vi "Configure.vi"(6 "GridSize":u32, 7 "Mode":u32, 8 "error in (no error)":errorcluster, 9 "Recording Settings":T1, 11 "AODAcq in":refnum<class "AODAcq.lvclass">) -> (0 "error out":errorcluster, 3 "AODAcq out":refnum<class "AODAcq.lvclass">)   [LabVIEW 2011, in "AODAcq.lvclass"]
uses:
  AODAcq.lvclass
  AODAcq.lvclass/AODAcq.ctl
  <instrlib>/niHWS/nihws.llb/niHWS Group String Attribute ID.ctl
  <instrlib>/niHWS/nihws.llb/niHWS Open File Permissions ID.ctl
  <vilib>/Utility/error.llb/Error Cluster From Error Code.vi
  Program Files/National Instruments/LabVIEW 2011/Targets/NI/FPGA/StockFPGA_IntfPrivate/ScriptTemplates/StockFPGA_PlugInRead32.vi
  <vilib>/rvi/errors/niLvFpgaAdjustHostInterfaceError.vi
  <instrlib>/niHWS/nihws.llb/niHWS Write Analog I16.vi
  <vilib>/rvi/interface/nirviReadWriteControl/nirviReadWriteControl.xnode
  FPGA_Control/AODRef.ctl
  FPGA_Control/FPGA Bitfiles/AODControl_FPGATarget_5751Acquire_F1CF9257.lvbitx
  FPGA_Control/AOD Control (FPGA).vi
  NiFpgaLv.dll
  <vilib>/FPGAPlugInAG/PXIe-7965R/niLvFpga_Read32_PXIe-7965R.vi
  <vilib>/rvi/interface/nirviReadWriteControl/niFpgaRWControlAccessTimeoutTemplate.vi
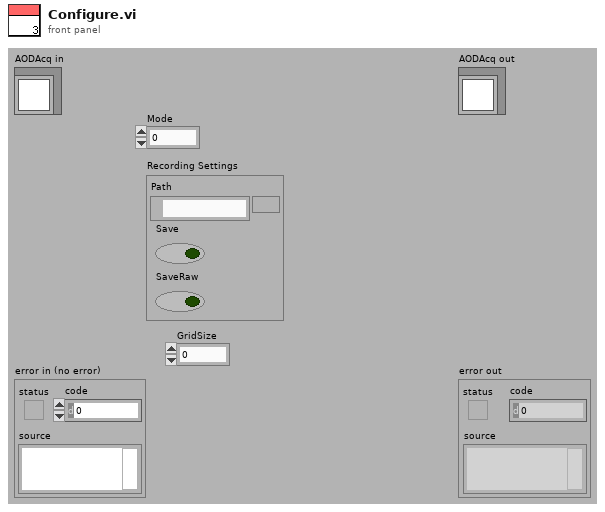
[diagram p1: front panel]
types:
  T1 = cluster{"Path":path, "Save":bool, "SaveRaw":bool}
  T2 = typedef "niHWS Open File Permissions ID.ctl" = enum32{"Read Only", "Read/Write Existing", "Read/Write/Create New", "Read/Write/Create New Always"}
  T3 = typedef "AODRef.ctl" = refnum<k20>
  T4 = typedef "niHWS Group String Attribute ID.ctl" = enum32{"Note", "Technician", "Project", "Timestamp"}
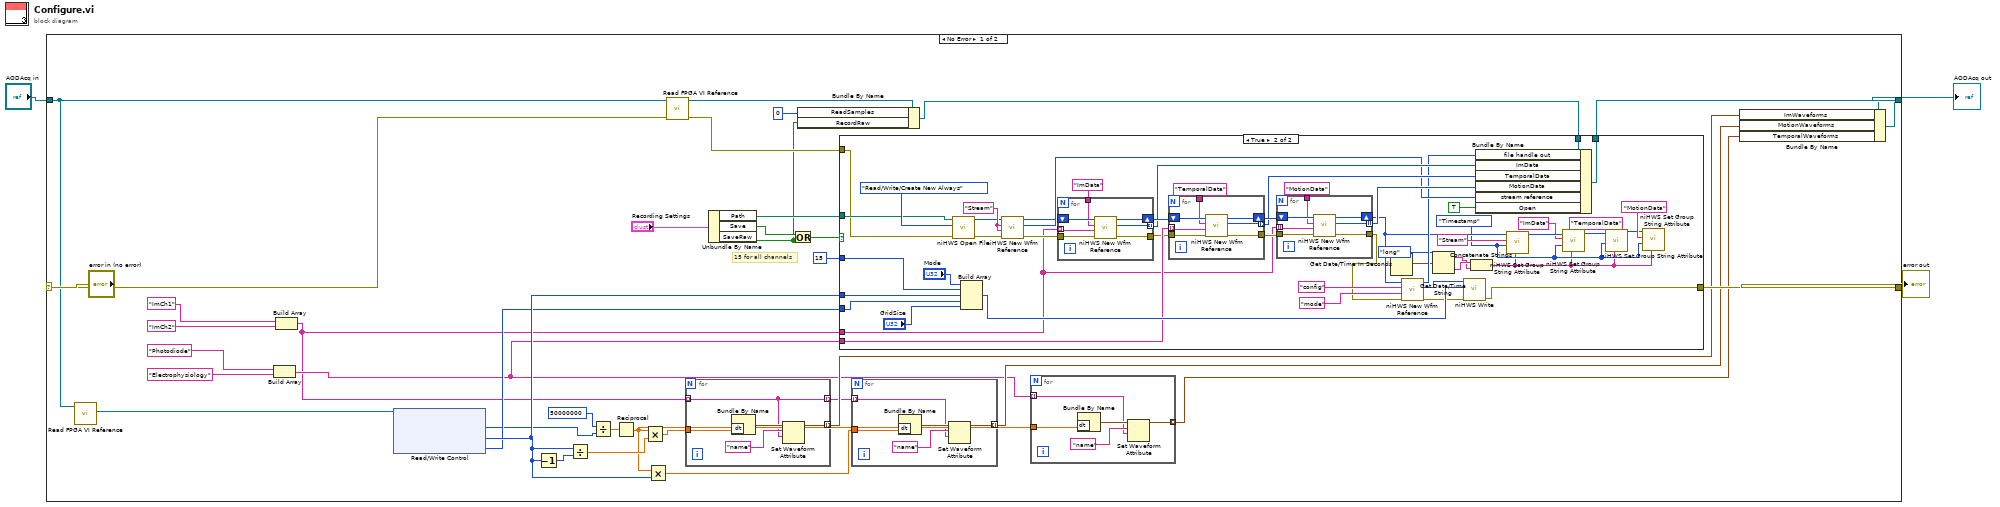
[diagram p0: block diagram]
diagram:
  n1 = case shown="No Error" "error in (no error)" {
    selector: "error in (no error)" -> [w11 w131]
    tunnel: [w36 w131] -> w3
    tunnel: [w26 w130] -> w1
    tunnel: "AODAcq in" -> [w12 w130]
    frame No Error {
      # "15 for all channels"
      n2 = call-dynamic "Read FPGA VI Reference.vi"("AODAcq in"=w12) -> ("FPGA VI Reference"=w29:T3)  [unwired: 8 in, 2 out]
      n3 = Build Array("Photodiode", "Electrophysiology") -> (w10:string[])
      n4 = Build Array("ImCh1", "ImCh2") -> (w9:string[])
      n5 = xnode "Read/Write Control"("FPGA VI Reference In"=w29) -> ("Setup.Downsample"=w5:u32, "Scan.Motion Increment"=w14:u32, "Scan.NumMotionPoints"=w13:u32)  [unwired: 1 in, 2 out]
      n6 = Decrement(x=w14) -> (x-1=w21:u32)
      n7 = Divide(x=w14, y=w21) -> (x/y=w20:dbl)
      n8 = Divide(x=50000000, y=w5) -> (x/y=w31:dbl)
      n9 = Reciprocal(x=w31) -> (1/x=w19:dbl)
      n10 = Multiply(x=w19, y=w20) -> (x*y=w22:dbl)
      n11 = Multiply(x=w19, y=w14) -> (x*y=w18:dbl)
      n12 = call-dynamic "Read FPGA VI Reference.vi"("error in (no error)"=w11, "AODAcq in"=w12) -> ("error out"=w24:errorcluster, "AODAcq out"=w25:refnum<class "AODAcq.lvclass">)  [unwired: 7 in, 1 out]
      n13 = for {
        tunnel: w9 -> [w51] mode=indexing
        tunnel: w22 -> [w55]
        tunnel: [w52] -> w28 mode=indexing
        tunnel: [w51] -> w17 mode=indexing
        n14 = Bundle By Name("dt"=w55) -> (w54:waveform(dbl))  [unwired: 1 in]
        n15 = Set Waveform Attribute(5:w51, 6:"name" ("name"), 7:w54) -> (3:w52:waveform(dbl))  [unwired: 1 in, 2 out]
      }
      n16 = Unbundle By Name("Recording Settings") -> ("Path"=w39:path, "Save"=w40:bool, "SaveRaw"=w23:bool)
      n17 = Or(x=w40, y=w23) -> (x .or. y?=w37:bool)
      n18 = Bundle By Name(cluster=w25, "ReadSamples"=u64 0, "RecordRaw"=w23) -> (w34:refnum<class "AODAcq.lvclass">)
      n19 = case shown="True" w37 {
        tunnel: w39 -> [_ w99]
        tunnel: w34 -> [w57 w95]
        tunnel: [w57 w94] -> w27
        tunnel: w24 -> [w56 w98]
        tunnel: [w56 w78] -> w36
        tunnel: w9 -> [_ w85]
        tunnel: w10 -> [_ w90]
        tunnel: w14 -> [_ w75]
        tunnel: w13 -> [_ w76]
        tunnel: u32 15 -> [_ w74]
        frame False {
        }
        frame True {
          w60 = niHWS_Group_String_Attribute_ID."Timestamp" ("attribute ID")
          w105 = "Stream" ("group name (empty)")
          n20 = call <instrlib>:"niHWS Open File.vi"("error in (no error)"=w98, "permissions (0:read only)"=niHWS_Open_File_Permissions_ID."Read/Write/Create New Always", "file path"=w99) -> ("error out"=w104:errorcluster, "file handle"=w93:u32)  [unwired: 7 in]
          n21 = Build Array("Mode", w74, w75, w76, "GridSize") -> (w101:u32[])
          n22 = call <instrlib>:"niHWS New Wfm Reference.vi"("error in (no error)"=w104, "waveform name (empty)"=w105, "group name (empty)"=w105, "file handle in"=w93) -> ("error out"=w103:errorcluster, "waveform reference"=w80:u32, "file handle out"=w73:u32)  [unwired: 5 in]
          n23 = for {
            tunnel: w103 -> [w127]
            tunnel: [w126] -> w88
            tunnel: "ImData" ("group name (empty)") -> [w125]
            tunnel: w85 -> [w124] mode=indexing
            shift-right: [w129] -> w91
            shift-left: w73 -> [w128]
            tunnel: [w123] -> w83 mode=indexing
            n24 = call <instrlib>:"niHWS New Wfm Reference.vi"("error in (no error)"=w127, "waveform name (empty)"=w124, "group name (empty)"=w125, "file handle in"=w128) -> ("error out"=w126:errorcluster, "waveform reference"=w123:u32, "file handle out"=w129:u32)  [unwired: 5 in]
          }
          n25 = for {
            tunnel: w88 -> [w120]
            tunnel: [w119] -> w87
            tunnel: "TemporalData" ("group name (empty)") -> [w118]
            tunnel: w90 -> [w117] mode=indexing
            shift-right: [w122] -> w86
            shift-left: w91 -> [w121]
            tunnel: [w116] -> w82 mode=indexing
            n26 = call <instrlib>:"niHWS New Wfm Reference.vi"("error in (no error)"=w120, "waveform name (empty)"=w117, "group name (empty)"=w118, "file handle in"=w121) -> ("error out"=w119:errorcluster, "waveform reference"=w116:u32, "file handle out"=w122:u32)  [unwired: 5 in]
          }
          n27 = for {
            tunnel: w87 -> [w113]
            tunnel: [w112] -> w79
            tunnel: "MotionData" ("group name (empty)") -> [w111]
            tunnel: w85 -> [w110] mode=indexing
            shift-right: [w115] -> w72
            shift-left: w86 -> [w114]
            tunnel: [w109] -> w81 mode=indexing
            n28 = call <instrlib>:"niHWS New Wfm Reference.vi"("error in (no error)"=w113, "waveform name (empty)"=w110, "group name (empty)"=w111, "file handle in"=w114) -> ("error out"=w112:errorcluster, "waveform reference"=w109:u32, "file handle out"=w115:u32)  [unwired: 5 in]
          }
          n29 = Get Date/Time In Seconds() -> (seconds since 1Jan1904=w70:timestamp)
          n30 = call <instrlib>:"niHWS New Wfm Reference.vi"("error in (no error)"=w79, "waveform name (empty)"="mode", "group name (empty)"="config", "file handle in"=w72) -> ("error out"=w100:errorcluster, "waveform reference"=w106:u32, "file handle out"=w77:u32)  [unwired: 5 in]
          n31 = Get Date/Time String(date format (0)=enum16{"short", "long", "abbreviated"}."long", seconds (now)=w70) -> (date string=w67:string, time string=w68:string)  [unwired: 1 in]
          n32 = call-poly <instrlib>:"niHWS Write.vi"("error in (no error)"=w100, "data"=w101, "waveform reference in"=w106) -> ("error out"=w78:errorcluster)  [unwired: 7 in, 1 out]
          n33 = Concatenate Strings(w68, w67) -> (w59:string)
          n34 = Bundle By Name(cluster=w95, "file handle out"=w77, "ImData"=w83, "TemporalData"=w82, "MotionData"=w81, "stream reference"=w80, "Open"=TRUE) -> (w94:refnum<class "AODAcq.lvclass">)
          n35 = call <instrlib>:"niHWS Set Group String Attribute.vi"("attribute value"=w59, "attribute ID"=w60, "group name (empty)"="Stream", "file handle in"=w72) -> ("file handle out"=w66:u32)  [unwired: 6 in, 1 out]
          n36 = call <instrlib>:"niHWS Set Group String Attribute.vi"("attribute value"=w59, "attribute ID"=w60, "group name (empty)"="ImData", "file handle in"=w66) -> ("file handle out"=w64:u32)  [unwired: 6 in, 1 out]
          n37 = call <instrlib>:"niHWS Set Group String Attribute.vi"("attribute value"=w59, "attribute ID"=w60, "group name (empty)"="TemporalData", "file handle in"=w64) -> ("file handle out"=w61:u32)  [unwired: 6 in, 1 out]
          n38 = call <instrlib>:"niHWS Set Group String Attribute.vi"("attribute value"=w59, "attribute ID"=w60, "group name (empty)"="MotionData", "file handle in"=w61) -> ()  [unwired: 6 in, 2 out]
        }
      }
      n39 = for {
        tunnel: w17 -> [w42] mode=indexing
        tunnel: w18 -> [w45]
        tunnel: [w41] -> w15 mode=indexing
        n40 = Bundle By Name("dt"=w45) -> (w44:waveform(dbl))  [unwired: 1 in]
        n41 = Set Waveform Attribute(5:w42, 6:"name" ("name"), 7:w44) -> (3:w41:waveform(dbl))  [unwired: 1 in, 2 out]
      }
      n42 = for {
        tunnel: w10 -> [w47] mode=indexing
        tunnel: w19 -> [w50]
        tunnel: [w46] -> w16 mode=indexing
        n43 = Bundle By Name("dt"=w50) -> (w49:waveform(dbl))  [unwired: 1 in]
        n44 = Set Waveform Attribute(5:w47, 6:"name" ("name"), 7:w49) -> (3:w46:waveform(dbl))  [unwired: 1 in, 2 out]
      }
      n45 = Bundle By Name(cluster=w27, "ImWaveforms"=w28, "MotionWaveforms"=w15, "TemporalWaveforms"=w16) -> (w26:refnum<class "AODAcq.lvclass">)
    }
    frame Error {
    }
  }
  "error out" <- w3
  "AODAcq out" <- w1
